vi "Stop Core.vi"(10 "final error code":i32, 11 "Test Executive Builder in":refnum<class "Test Executive Builder.lvclass">) -> (3 "Test Executive Builder out":refnum<class "Test Executive Builder.lvclass">)   [LabVIEW 2017, in "Test Executive Builder.lvclass"]
doc: "(<B>Filename</B>: Actor Framework.lvlib:Actor.lvclass:Stop Core.vi)\n\nDefines what the actor does before it stops. Use the <B>final error code</B> input to determine whether the actor shut down in response to an error.\n\nBy default, this method does nothing. A descendant class may override it to define behavior, such as shutting down any processes the actor initiated in its override of the Actor Core method."
uses:
  <vilib>/gpm_packages/@cs/Test-executive-builder/Example/Application/Test Executive Builder/Test Executive Builder/Test Executive Builder.lvclass
  <vilib>/gpm_packages/@cs/Test-executive-builder/Example/Application/Test Executive Builder/Test Executive Builder/Test Executive Builder.lvclass/Test Executive Builder.ctl
  <vilib>/ActorFramework/Message Enqueuer/Message Enqueuer.lvclass/Message Enqueuer.ctl
  <vilib>/ActorFramework/Message Enqueuer/Enqueue.vi
  <vilib>/ActorFramework/Stop Msg/Stop Msg.lvclass
  C:/Program Files/National Instruments/LabVIEW 2017/vi.lib/ActorFramework/Message/Message.lvclass
  <vilib>/ActorFramework/Message Priority Queue/Priority Enqueue.vi
  <vilib>/gpm_packages/@cs/Test-executive-builder/Source/Test Executive Builder Model/Test Executive Builder Model/Test Executive Builder Model.lvclass
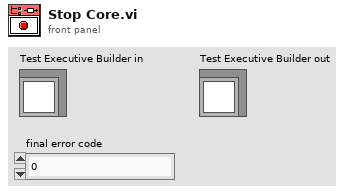
[diagram p1: front panel]
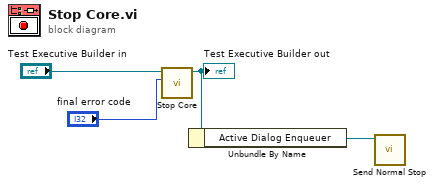
[diagram p0: block diagram]
diagram:
  n1 = call-parent "Stop Core.vi"("final error code"="final error code", "IObserver in"="Test Executive Builder in") -> ("IObserver out"=w2:refnum<class "Test Executive Builder.lvclass">)  [unwired: 9 in]
  "Test Executive Builder out" <- w2
  n2 = Unbundle By Name(w2) -> ("Active Dialog Enqueuer"=w1:refnum<class "Message Enqueuer.lvclass">)
  n3 = call <vilib>:"Send Normal Stop.vi"("Message Enqueuer"=w1) -> ()  [unwired: 10 in, 1 out]
